vi "createCheese.vi"(8 "error in (no error)":errorcluster, 11 "PizzaIngredientFactory in":refnum<class "PizzaIngredientFactory.lvclass">) -> (0 "error out":errorcluster, 2 "Ingredients":string, 3 "PizzaIngredientFactory out":refnum<class "PizzaIngredientFactory.lvclass">)   [LabVIEW 2013, in "PizzaIngredientFactory.lvclass"]
uses:
  PizzaIngredientFactory.lvclass
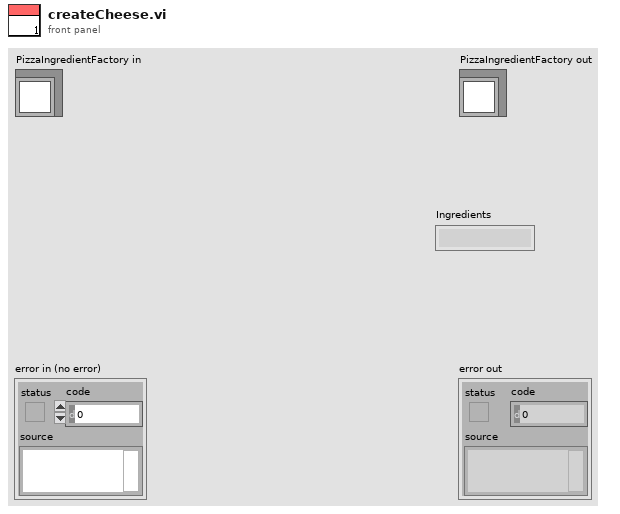
[diagram p1: front panel]
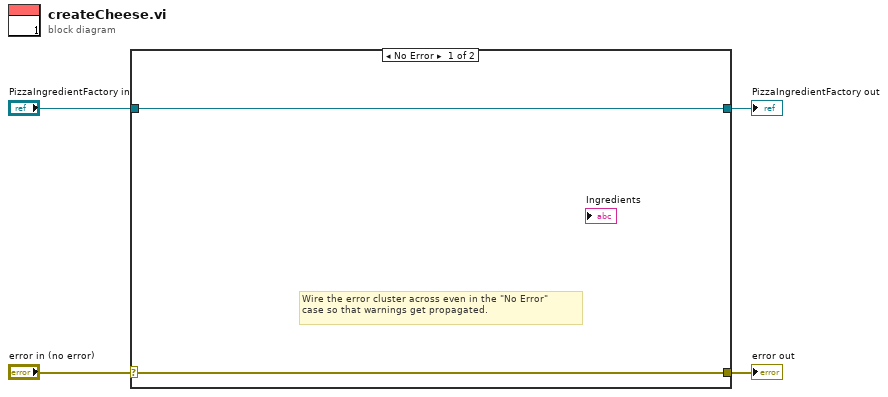
[diagram p0: block diagram]
diagram:
  n1 = case shown="No Error" "error in (no error)" {
    selector: "error in (no error)" -> [w5 w8]
    tunnel: [w5 w8] -> w3
    tunnel: [w6 w7] -> w1
    tunnel: "PizzaIngredientFactory in" -> [w6 w7]
    frame No Error {
      # "Wire the error cluster across even in the \"No Error\"\ncase so that warnings get propagated."
    }
    frame Error {
    }
  }
  "error out" <- w3
  "PizzaIngredientFactory out" <- w1
